vi "daqio_Data_Buffer_FGV.vi"(4 "Is Array?":bool, 6 "Buffer Settings":T1={"Max File Size (Bytes)"=100, "Save File after no of Writes"=1000000, "Timeout"=10000}, 7 "Buffer Command":T3, 8 "error in (no error)":errorcluster, 9 "JSON Data":string, 10 "API route":string="TimeSeriesEntries", 11 "daq.io type in":T4={"daq.io ref"=refnum, "daq.io API Base"="", "Device Key"="", "Account ID"="", "online"=TRUE, "SSL"=FALSE}) -> (0 "error out":errorcluster, 3 "daq.io type out":T4={"daq.io ref"=refnum, "daq.io API Base"="", "Device Key"="", "Account ID"="", "online"=TRUE, "SSL"=FALSE})   [LabVIEW 2013, in "daqio minimal.lvlib"]
doc: "When offline, this VI accepts the current data to be posted, stores it in human-readable text files and makes sure not too much data will be buffered that could cause issues when the connection resumes at a later point. \n\nThe \"Is Array\" flag needs to be set in functions that post arrays of data, so it will be correctly written into the buffer file."
uses:
  daqio minimal.lvlib
  _typedefs/daqio-Type.ctl
  <vilib>/httpClient/ClientHandle.ctl
  _typedefs/daqio-Buffer-Commands.ctl
  _typedefs/daqio-Buffer-Cluster.ctl
  _typedefs/daqio-Buffer-Parameters.ctl
  _typedefs/connection_FGV_commands.ctl
  <vilib>/Easy HTTP Client/Easy HTTP.lvlib
  <vilib>/httpClient/LabVIEWHTTPClient.lvlib
panel:
  out "All buffer files":T2[](array[typedef])
  out "Buffer empty":bool
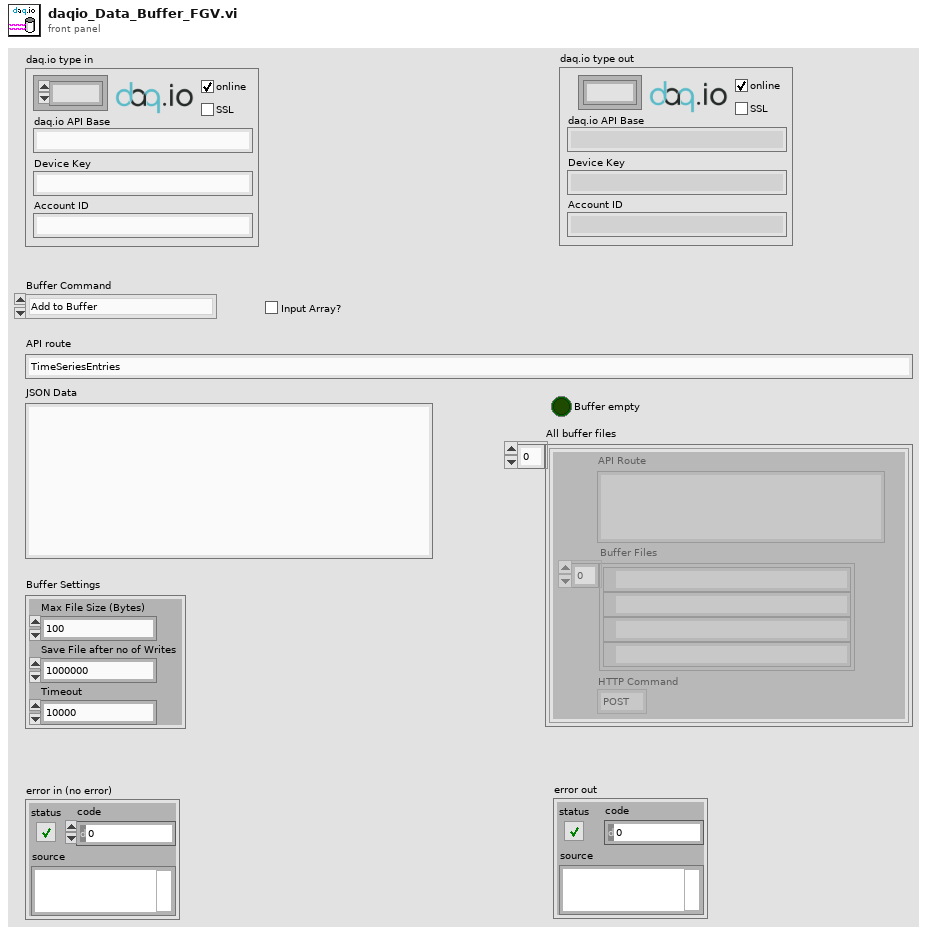
[diagram p1: front panel]
types:
  T1 = typedef "daqio minimal.lvlib/daqio-Buffer-Parameters.ctl" = cluster{"Max File Size (Bytes)":i32, "Save File after no of Writes":i32, "Timeout":i32}
  T2 = typedef "daqio minimal.lvlib/daqio-Buffer-Cluster.ctl" = cluster{"API Route":string, "Buffer Files":path[], "HTTP Command":enum16{"POST", "PUT"}}
  T3 = typedef "daqio minimal.lvlib/daqio-Buffer-Commands.ctl" = enum16{"Add to Buffer", "Post from Buffer", "Clear Buffer", "Init"}
  T4 = typedef "daqio minimal.lvlib/daqio-Type.ctl" = cluster{"daq.io ref":T5, "daq.io API Base":string, "Device Key":string, "Account ID":string, "online":bool, "SSL":bool}
  T5 = typedef "LabVIEWHTTPClient.lvlib/ClientHandle.ctl" = refnum<k1>
  T6 = typedef "daqio minimal.lvlib/connection_FGV_commands.ctl" = enum16{"Set Conn Stat", "Save Type", "Get Type from File", "Set Type", "Set Buffer", "Get"}
  T7 = enum16{"open", "replace", "create", "open or create", "replace or create", "replace or create with confirmation"}
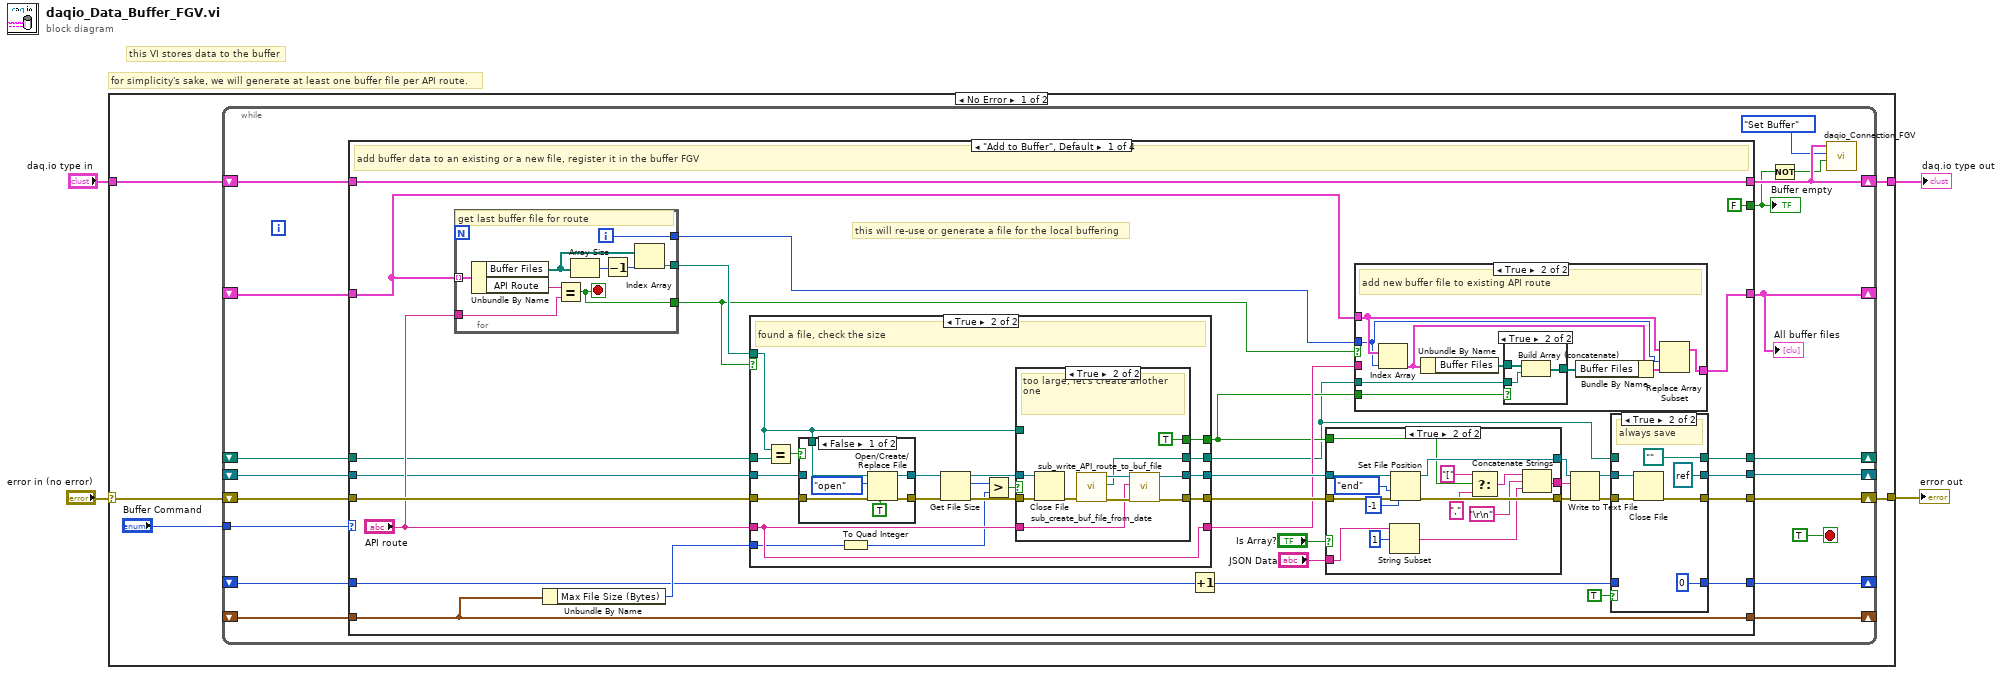
[diagram p0: block diagram]
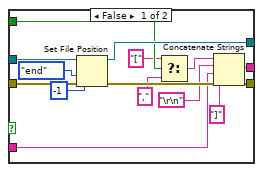
[diagram p2: hidden frame]
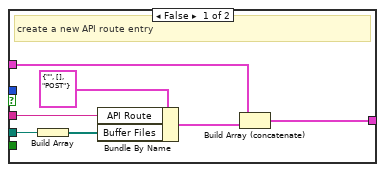
[diagram p4: hidden frame]
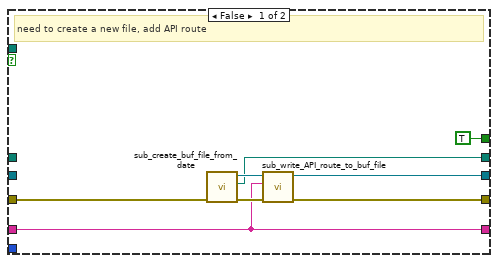
[diagram p6: hidden frame]
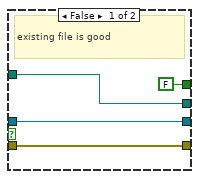
[diagram p8: hidden frame]
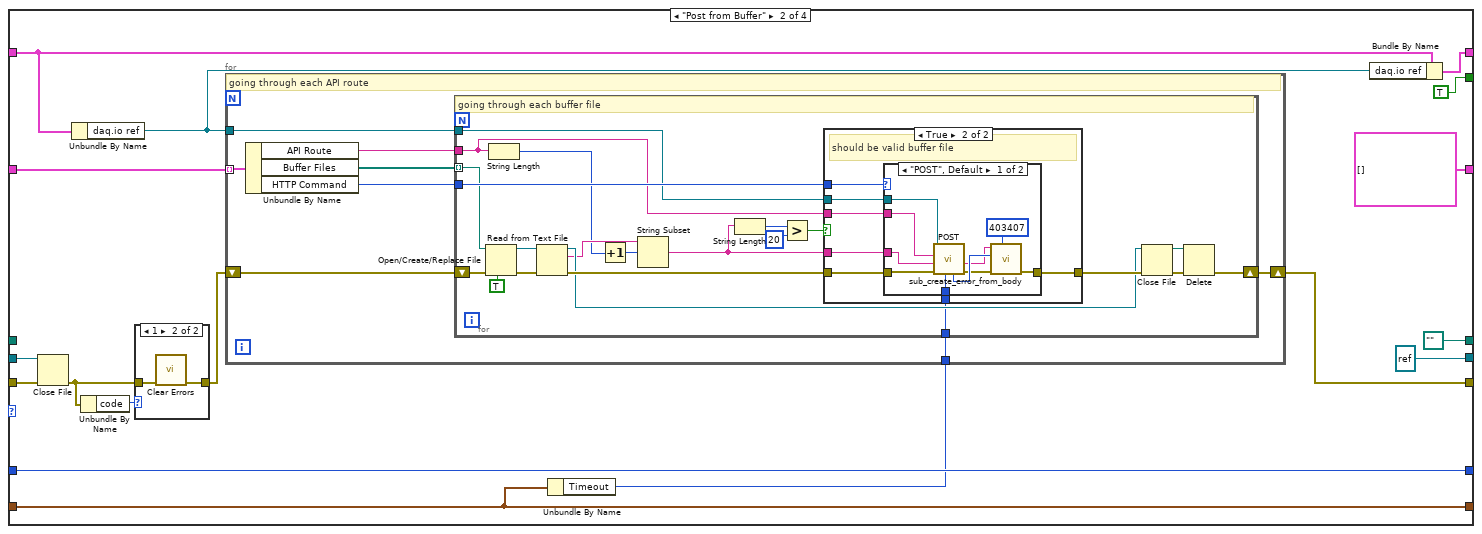
[diagram p9: hidden frame]
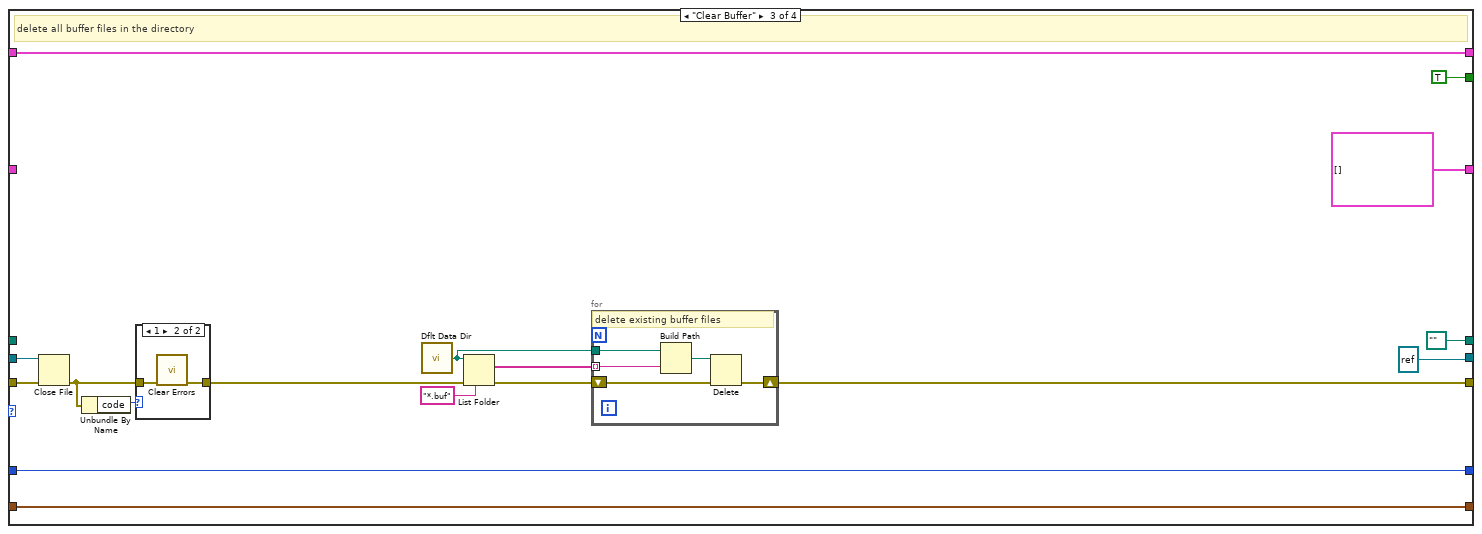
[diagram p13: hidden frame]
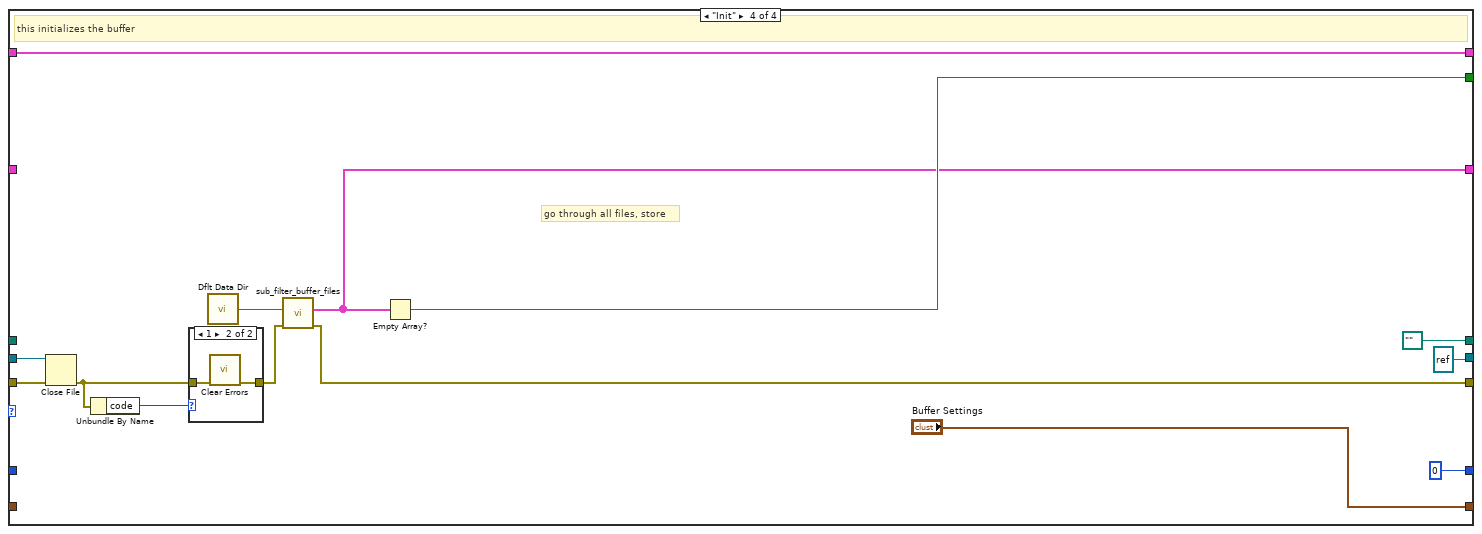
[diagram p15: hidden frame]
diagram:
  # "for simplicity's sake, we will generate at least one buffer file per API route."
  # "this VI stores data to the buffer"
  n1 = case shown="No Error" "error in (no error)" {
    selector: "error in (no error)" -> [w7 w288]
    tunnel: "daq.io type in" -> [w9 w289]
    tunnel: [w6 w288] -> w2
    tunnel: [w5 w289] -> w3
    frame No Error {
      n2 = while {
        shift-right: [w13] -> w5
        shift-left: w9 -> [w22]
        tunnel: "Buffer Command" -> [w27]
        shift-right: [w25] -> w6
        shift-left: w7 -> [w26]
        shift-right: [w23] -> _
        shift-left: _ -> [w24]
        shift-right: [w21] -> _
        shift-left: _ -> [w20]
        shift-right: [w19] -> _
        shift-left: _ -> [w18]
        shift-right: [w17] -> _
        shift-left: _ -> [w16]
        shift-right: [w15] -> _
        shift-left: _ -> [w14]
        stop <- TRUE stop-if-true
        n3 = case shown="\"Add to Buffer\", Default" w27 {
          tunnel: w26 -> [w55 w187 w248 w277]
          tunnel: [w57 w184 w262 w281] -> w25
          tunnel: [FALSE TRUE TRUE w284] -> w10
          tunnel: [w51 T2[] [] ("Output Routes and Files") T2[] [] ("Output Routes and Files") w282] -> w23
          tunnel: w24 -> [w32 w189 _ _]
          tunnel: w22 -> [w49 w191 w255 w280]
          tunnel: [w49 w190 w255 w280] -> w13
          tunnel: [w38 w178 w254 "Buffer Settings"] -> w21
          tunnel: w20 -> [w38 w178 w254 _]
          tunnel: [w41 refnum<file> refnum ("refnum out") refnum<file> refnum ("refnum out") refnum<file> refnum ("refnum out")] -> w19
          tunnel: w18 -> [w44 w188 w247 w278]
          tunnel: [w39 path "" ("new file path") path "" ("new file path") path "" ("new file path")] -> w17
          tunnel: w16 -> [w43 _ _ _]
          tunnel: [w35 w192 w253 0] -> w15
          tunnel: w14 -> [w36 w192 w253 _]
          frame "Add to Buffer", Default {
            # "this will re-use or generate a file for the local buffering"
            # "add buffer data to an existing or a new file, register it in the buffer FGV"
            n4 = for {
              tunnel: w32 -> [w176] mode=indexing
              tunnel: "API route" -> [w174]
              tunnel: [w170] -> w54
              tunnel: [w169] -> w33
              tunnel: [w168] -> w31
              i -> [w168]
              stop <- w169 stop-if-true
              # "get last buffer file for route"
              n5 = Unbundle By Name(w176) -> ("Buffer Files"=w173:path[], "API Route"=w175:string)
              n6 = Equal?(x=w175, y=w174) -> (x = y?=w169:bool)
              n7 = Array Size(array=w173) -> (size(s)=w172:i32)
              n8 = Decrement(x=w172) -> (x-1=w171:i32)
              n9 = Index Array(array=w173, index=w171) -> (element=w170:path)
            }
            n10 = Unbundle By Name(w38) -> ("Max File Size (Bytes)"=w37:i32)
            n11 = case shown="True" w33 {
              tunnel: w55 -> [w127 w145]
              tunnel: w54 -> [_ w132]
              tunnel: "API route" -> [w121 w135]
              tunnel: [w124 w138] -> w53
              tunnel: [w123 w137] -> w52
              tunnel: [w122 w136] -> w40
              tunnel: [w121 w135] -> w50
              tunnel: [TRUE w134] -> w45
              tunnel: w44 -> [_ w130]
              tunnel: w43 -> [_ w133]
              tunnel: w37 -> [_ w129]
              frame False {
                # "need to create a new file, add API route"
                n12 = call "sub_create_buf_file_from_date.vi"("error in (no error)"=w127) -> ("error out"=w126:errorcluster, "new file path"=w122:path, "File Refnum"=w125:refnum<file>)  [unwired: 8 in]
                n13 = call "sub_write_API_route_to_buf_file.vi"("error in (no error)"=w126, "API route"=w121, "Buffer File in"=w125) -> ("error out"=w123:errorcluster, "Buffer File out"=w124:refnum<file>)  [unwired: 7 in]
              }
              frame True {
                # "found a file, check the size"
                n14 = Equal?(x=w132, y=w133) -> (x = y?=w131:bool)
                n15 = case shown="False" w131 {
                  tunnel: w145 -> [w150 w152]
                  tunnel: [w149 w152] -> w144
                  tunnel: [w148 w153] -> w143
                  tunnel: w132 -> [w147 _]
                  tunnel: w130 -> [_ w153]
                  frame False {
                    n16 = Open/Create/Replace File(file path (use dialog)=w147, error in=w150, operation (0:open)=T7."open", disable buffering (F)=TRUE) -> (refnum out=w148:refnum<file>, error out=w149:errorcluster)  [unwired: 2 in, 1 out]
                  }
                  frame True {
                  }
                }
                n17 = To Quad Integer(1:w129) -> (0:w128:i64)
                n18 = Get File Size(file=w143, error in=w144) -> (refnum out=w139:refnum<file>, size (in bytes)=w142:i64, 0:w140:errorcluster)
                n19 = Greater?(x=w142, y=w128) -> (0:w141:bool)
                n20 = case shown="True" w141 {
                  tunnel: w140 -> [w156 w167]
                  tunnel: w139 -> [w157 w166]
                  tunnel: [w157 w162] -> w138
                  tunnel: [w156 w163] -> w137
                  tunnel: w135 -> [_ w160]
                  tunnel: [w155 w159] -> w136
                  tunnel: w132 -> [w155 _]
                  tunnel: [FALSE TRUE] -> w134
                  frame False {
                    # "existing file is good"
                  }
                  frame True {
                    # "too large, let's create another one"
                    n21 = Close File(refnum=w166, error in=w167) -> (error out=w165:errorcluster)  [unwired: 1 out]
                    n22 = call "sub_create_buf_file_from_date.vi"("error in (no error)"=w165) -> ("error out"=w164:errorcluster, "new file path"=w159:path, "File Refnum"=w161:refnum<file>)  [unwired: 8 in]
                    n23 = call "sub_write_API_route_to_buf_file.vi"("error in (no error)"=w164, "API route"=w160, "Buffer File in"=w161) -> ("error out"=w163:errorcluster, "Buffer File out"=w162:refnum<file>)  [unwired: 7 in]
                  }
                }
              }
            }
            n24 = Increment(x=w36) -> (x+1=w34:i32)
            n25 = case shown="True" "Is Array?" {
              tunnel: [w74 w89] -> w59
              tunnel: [w73 w88] -> w58
              tunnel: w53 -> [w71 w86]
              tunnel: w52 -> [w70 w85]
              tunnel: [w67 w82] -> w47
              tunnel: "JSON Data" -> [w64 w76]
              tunnel: w45 -> [w63 w79]
              frame False {
                n26 = Set File Position(offset (in bytes) (0)=i64 -1, refnum=w71, from (0:start)=enum16{"start", "end", "current"}."end", error in=w70) -> (refnum out=w74:refnum<file>, error out=w73:errorcluster)
                n27 = Select(t="[", s=w63, f="," ("string")) -> (s? t:f=w66:string)
                n28 = Concatenate Strings(w66, "\r\n", w64, "]" ("string")) -> (w67:string)
              }
              frame True {
                n29 = String Subset(string=w76, offset (0)=1) -> (substring=w75:string)  [unwired: 1 in]
                n30 = Set File Position(offset (in bytes) (0)=i64 -1, refnum=w86, from (0:start)=enum16{"start", "end", "current"}."end", error in=w85) -> (refnum out=w89:refnum<file>, error out=w88:errorcluster)
                n31 = Select(t="[", s=w79, f="," ("string")) -> (s? t:f=w81:string)
                n32 = Concatenate Strings(w81, "\r\n", w75) -> (w82:string)
              }
            }
            n33 = case shown="True" w33 {
              tunnel: w32 -> [w106 w110]
              tunnel: [w100 w115] -> w51
              tunnel: w40 -> [w104 w113]
              tunnel: w50 -> [w102 _]
              tunnel: w45 -> [_ w108]
              tunnel: w31 -> [_ w107]
              frame False {
                # "create a new API route entry"
                n34 = Build Array(w104) -> (w103:path[])
                n35 = Bundle By Name(cluster=T2 {"API Route"="", "Buffer Files"=[], "HTTP Command"=enum."POST"} ("element"), "API Route"=w102, "Buffer Files"=w103) -> (w101:T2)
                n36 = Build Array (concatenate)(w106, w101) -> (w100:T2[])
              }
              frame True {
                # "add new buffer file to existing API route"
                n37 = Index Array(array=w110, index=w107) -> (element=w111:T2)
                n38 = Unbundle By Name(w111) -> ("Buffer Files"=w114:path[])
                n39 = case shown="True" w108 {
                  tunnel: w114 -> [w116 w119]
                  tunnel: w113 -> [_ w118]
                  tunnel: [w116 w117] -> w112
                  frame False {
                  }
                  frame True {
                    n40 = Build Array (concatenate)(w119, w118) -> (w117:path[])
                  }
                }
                n41 = Bundle By Name(cluster=w111, "Buffer Files"=w112) -> (w109:T2)
                n42 = Replace Array Subset(array=w110, new element=w109, index=w107) -> (w115:T2[])
              }
            }
            n43 = Write to Text File(file (use dialog)=w59, text=w47, error in=w58) -> (refnum out=w42:refnum<file>, error out=w60:errorcluster)  [unwired: 1 in, 1 out]
            n44 = case shown="True" TRUE {
              tunnel: w60 -> [w93 w99]
              tunnel: [w93 w98] -> w57
              tunnel: w42 -> [w92 w97]
              tunnel: [w92 refnum<file> refnum ("refnum out")] -> w41
              tunnel: w40 -> [w91 _]
              tunnel: [w91 path "" ("new file path")] -> w39
              tunnel: [w90 0] -> w35
              tunnel: w34 -> [w90 _]
              frame False {
              }
              frame True {
                # "always save"
                n45 = Close File(refnum=w97, error in=w99) -> (error out=w98:errorcluster)  [unwired: 1 out]
              }
            }
          }
          frame "Post from Buffer" {
            n46 = Close File(refnum=w188, error in=w187) -> (error out=w179:errorcluster)  [unwired: 1 out]
            n47 = Unbundle By Name(w191) -> ("daq.io ref"=w183:T5)
            n48 = Unbundle By Name(w179) -> ("code"=w181:i32)
            n49 = case shown="1" w181 {
              tunnel: [w194 w196] -> w180
              tunnel: w179 -> [w194 w195]
              frame 0, Default {
              }
              frame 1 {
                n50 = call <vilib>:"Clear Errors.vi"("error in (no error)"=w195) -> ("error out"=w196:errorcluster)  [unwired: 6 in]
              }
            }
            n51 = Unbundle By Name(w178) -> ("Timeout"=w177:i32)
            n52 = for {
              tunnel: w189 -> [w204] mode=indexing
              shift-right: [w201] -> w184
              shift-left: w180 -> [w202]
              tunnel: w183 -> [w198]
              tunnel: w177 -> [w197]
              # "going through each API route"
              n53 = Unbundle By Name(w204) -> ("API Route"=w199:string, "Buffer Files"=w203:path[], "HTTP Command"=w200:enum16{"POST", "PUT"})
              n54 = for {
                tunnel: w203 -> [w224] mode=indexing
                shift-right: [w216] -> w201
                shift-left: w202 -> [w225]
                tunnel: w200 -> [w226]
                tunnel: w199 -> [w213]
                tunnel: w198 -> [w211]
                tunnel: w197 -> [w210]
                # "going through each buffer file"
                n55 = Open/Create/Replace File(file path (use dialog)=w224, error in=w225, disable buffering (F)=TRUE) -> (refnum out=w222:refnum<file>, error out=w223:errorcluster)  [unwired: 3 in, 1 out]
                n56 = String Length(string=w213) -> (length=w214:i32)
                n57 = Read from Text File(file (use dialog)=w222, error in=w223) -> (refnum out=w219:refnum<file>, text=w215:string, error out=w221:errorcluster)  [unwired: 2 in, 1 out]
                n58 = Increment(x=w214) -> (x+1=w212:i32)
                n59 = String Subset(string=w215, offset (0)=w212) -> (substring=w208:string)  [unwired: 1 in]
                n60 = String Length(string=w208) -> (length=w207:i32)
                n61 = Greater?(x=w207, y=20) -> (0:w205:bool)
                n62 = case shown="True" w205 {
                  tunnel: w226 -> [_ w234]
                  tunnel: w221 -> [w227 w233]
                  tunnel: [w227 w232] -> w220
                  tunnel: w213 -> [_ w231]
                  tunnel: w211 -> [_ w230]
                  tunnel: w210 -> [_ w229]
                  tunnel: w208 -> [_ w228]
                  frame False {
                    # "seems to be broken buffer file, delete it"
                  }
                  frame True {
                    # "should be valid buffer file"
                    n63 = case shown="\"POST\", Default" w234 {
                      tunnel: w233 -> [w243 w245]
                      tunnel: [w238 w245] -> w232
                      tunnel: w228 -> [w236 _]
                      tunnel: w231 -> [w237 _]
                      tunnel: w230 -> [w235 _]
                      tunnel: w229 -> [w244 _]
                      frame "POST", Default {
                        n64 = call <vilib>:"POST.vi"("timeout (10000)"=w244, "error in (no error)"=w243, "data"=w236, "url"=w237, "client handle"=w235) -> ("error out"=w241:errorcluster, "body"=w240:string, "HTTP Response Code"=w242:i32)  [unwired: 2 in, 2 out]
                        n65 = call "sub_create_error_from_body.vi"("error code"=403407, "error in (no error)"=w241, "http code"=w242, "body"=w240) -> ("error out"=w238:errorcluster)  [unwired: 7 in]
                      }
                      frame "PUT" {
                      }
                    }
                  }
                }
                n66 = Close File(refnum=w219, error in=w220) -> (path=w217:path, error out=w218:errorcluster)
                n67 = Delete(path (use dialog)=w217, error in=w218) -> (error out=w216:errorcluster)  [unwired: 3 in, 2 out]
              }
            }
            n68 = Bundle By Name(cluster=w191, "daq.io ref"=w183) -> (w190:T4)
          }
          frame "Clear Buffer" {
            # "delete all buffer files in the directory"
            n69 = Close File(refnum=w247, error in=w248) -> (error out=w249:errorcluster)  [unwired: 1 out]
            n70 = Unbundle By Name(w249) -> ("code"=w250:i32)
            n71 = case shown="1" w250 {
              tunnel: [w263 w265] -> w246
              tunnel: w249 -> [w263 w264]
              frame 0, Default {
              }
              frame 1 {
                n72 = call <vilib>:"Clear Errors.vi"("error in (no error)"=w264) -> ("error out"=w265:errorcluster)  [unwired: 6 in]
              }
            }
            n73 = call <vilib>:"Dflt Data Dir.vi"() -> ("App:Default Data Directory"=w256:path)
            n74 = List Folder(path=w256, pattern="*.buf", error in=w246) -> (filenames=w257:string[], error out=w258:errorcluster)  [unwired: 1 in, 2 out]
            n75 = for {
              shift-right: [w269] -> w262
              shift-left: w258 -> [w270]
              tunnel: w257 -> [w266] mode=indexing
              tunnel: w256 -> [w267]
              # "delete existing buffer files"
              n76 = Build Path(base path=w267, name or relative path=w266) -> (appended path=w268:path)
              n77 = Delete(path (use dialog)=w268, error in=w270) -> (error out=w269:errorcluster)  [unwired: 3 in, 2 out]
            }
          }
          frame "Init" {
            # "go through all files, store"
            # "this initializes the buffer"
            n78 = Close File(refnum=w278, error in=w277) -> (error out=w273:errorcluster)  [unwired: 1 out]
            n79 = Unbundle By Name(w273) -> ("code"=w274:i32)
            n80 = case shown="1" w274 {
              tunnel: [w285 w286] -> w272
              tunnel: w273 -> [w285 w287]
              frame 0, Default {
              }
              frame 1 {
                n81 = call <vilib>:"Clear Errors.vi"("error in (no error)"=w287) -> ("error out"=w286:errorcluster)  [unwired: 6 in]
              }
            }
            n82 = call <vilib>:"Dflt Data Dir.vi"() -> ("App:Default Data Directory"=w283:path)
            n83 = call "sub_filter_buffer_files.vi"("error in (no error)"=w272, "Start Folder"=w283) -> ("error out"=w281:errorcluster, "Output Routes and Files"=w282:T2[])  [unwired: 8 in]
            n84 = Empty Array?(array=w282) -> (empty?=w284:bool)
          }
        }
        "Buffer empty" <- w10
        "All buffer files" <- w23
        n85 = Not(x=w10) -> (.not. x?=w11:bool)
        n86 = call "daqio_Connection_FGV.vi"("Buffered Data exists"=w11, "Enum"=connection_FGV_commands."Set Buffer", "daq.io type in"=w13) -> ()  [unwired: 5 in, 4 out]
      }
    }
    frame Error {
    }
  }
  "error out" <- w2
  "daq.io type out" <- w3
